vi "Refresh.vi"(8 "error in (no error)":errorcluster, 10 "Force Refresh (F)":bool, 11 "BS120x in":refnum<class "BS120x.lvclass">) -> (0 "error out":errorcluster, 3 "BS120x out":refnum<class "BS120x.lvclass">)   [LabVIEW 2021, in "BS120x Driver.lvlib" / "BS120x.lvclass"]
uses:
  BS120x.lvclass
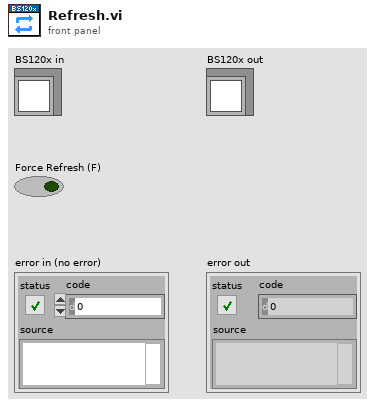
[diagram p1: front panel]
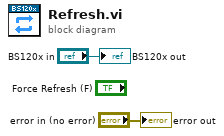
[diagram p0: block diagram]
diagram:
  "BS120x out" <- "BS120x in"
  "error out" <- "error in (no error)"
